vi "CI_StandardColorWrite.vi"(4 "error in (no error)":errorcluster, 5 "Value":u32(colorbox), 6 "Container State":T2, 7 "Display State In":T1={"StandardColor"=0, "WarningColor"=15671808, "CriticalColor"=15671808, "Standard<>Warning Range"=0, "Warning<>Critical Range"=0}) -> (0 "error out":errorcluster, 3 "Display State Out":T1={"StandardColor"=0, "WarningColor"=15671808, "CriticalColor"=15671808, "Standard<>Warning Range"=0, "Warning<>Critical Range"=0})   [LabVIEW 2010, in "CapacityIndicator.xctl"]
uses:
  CapacityIndicator.xctl
  <vilib>/_xctls/Container State.ctl
  CI_State.ctl
  <vilib>/_xctls/XControlSupport.lvlib
panel:
  # "Replace the Value Control below with a Control of desired type.\nDo not remove this Control or the others from the connector pane.\nDo not change the connector pane pattern.\nThe Value control should always be the third terminal from top on the input side in the connector pane."
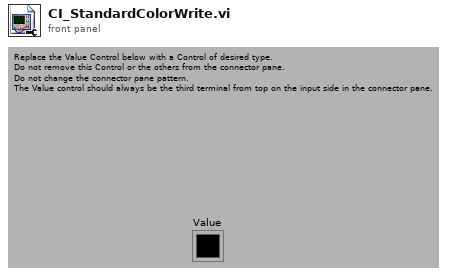
[diagram p1: front panel]
types:
  T1 = typedef "CapacityIndicator.xctl/CI_State.ctl" = cluster{"StandardColor":u32, "WarningColor":u32, "CriticalColor":u32, "Standard<>Warning Range":u8, "Warning<>Critical Range":u8}
  T2 = typedef "XControlSupport.lvlib/Container State.ctl" = cluster{"Indicator?":bool, "Run Mode?":bool, " Refnum":refnum<vi>}
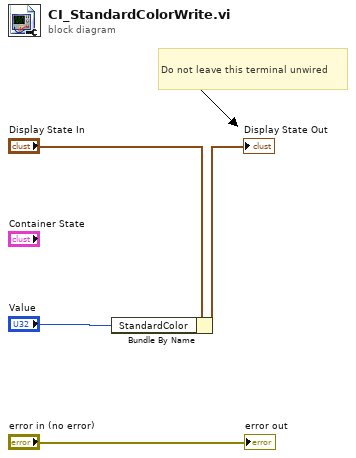
[diagram p0: block diagram]
diagram:
  # "Do not leave this terminal unwired"
  n1 = Bundle By Name(cluster="Display State In", "StandardColor"="Value") -> (→"Display State Out":T1)
  "error out" <- "error in (no error)"
